vi "Drag Drop Test.vi"() -> ()   [LabVIEW 2020]
uses:
  <vilib>/picture/picture.llb/imagedata.ctl
  <vilib>/event_ctls.llb/lveventtype.ctl
panel:
  out "2D Picture 3":picture
  out "2D Picture 2":picture
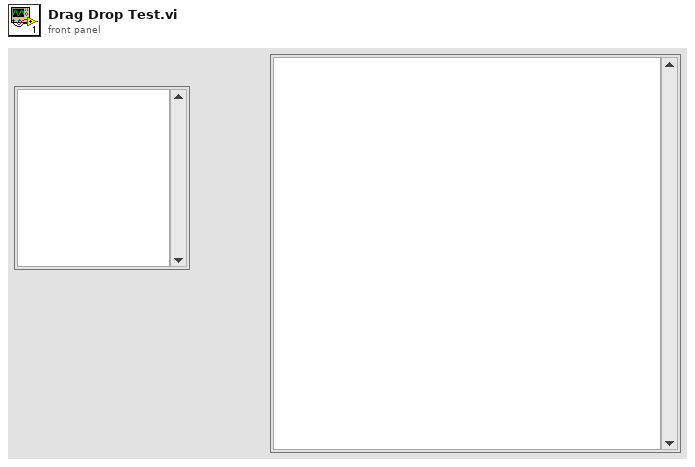
[diagram p1: front panel]
types:
  T1 = typedef "imagedata.ctl" = cluster{"image type":i32, "image depth":i32, "image":u8[], "mask":u8[], "colors":u32[], "Rectangle":cluster{"left":i16, "top":i16, "right":i16, "bottom":i16}}
  T2 = cluster{"Name":string, "CPTM.DataType":variant, "Get All Control Values Variant":cluster{"Name":string, "Variant Data":variant}[], "Color 256":T1}[]
  T3 = cluster{"left":i16, "top":i16, "right":i16, "bottom":i16}
  T4 = typedef "lveventtype.ctl" = enum32{"Null", "Timeout", "Annotation Menu Selection", "Annotation Menu Selection?", "App Instance Close", "App Instance Close?", "Autoscale Range Change", "Bookmark Info Change", "Cell Edit", "Cell Edit?", "Cursor Grab", "Cursor Grab?", "Cursor Menu Selection", "Cursor Menu Selection?", "Cursor Move", "Cursor Release", "Data Change", "Direction Change", "Display State Change", "Drag Ended", "Drag Enter", "Drag Leave", "Drag Over", "Drag Source Update", "Drag Starting", "Drag Starting?", "Drop", "Exec State Change", "Key Down", "Key Down?", "Key Repeat", "Key Repeat?", "Key Up", "Listbox Double Click", "Menu Activation?", "Menu Selection (App)", "Menu Selection? (App)", "Menu Selection (User)", "Mouse Down", "Mouse Down?", "Mouse Enter", "Mouse Leave", "Mouse Move", "Mouse Up", "Mouse Wheel", "NI Security User Change (App)", "Pane Size", "Panel Close", "Panel Close?", "Panel Resize", "Plot Attribute Change", "Scale Range Change", "Shortcut Menu Activation?", "Shortcut Menu Selection (App)", "Shortcut Menu Selection? (App)", "Shortcut Menu Selection (User)", "Tree Double Click", "Tree Drag", "Tree Drag?", "Tree Drop", "Tree Drop?", "Tree Item Close", "Tree Item Close?", "Tree Item Open", "Tree Item Open?", "User Event", "Value Change"}
  T5 = typedef "LVPoint32TypeDef.ctl" = cluster{"Horizontal":i32, "Vertical":i32}
  T6 = typedef "LVPointTypeDef.ctl" = cluster{"Horizontal":i16, "Vertical":i16}
  T7 = typedef "LVPositionTypeDef.ctl" = cluster{"Left":i32, "Top":i32}
  T8 = cluster{"Name":string, "CPTM.DataType":variant, "Get All Control Values Variant":cluster{"Name":string, "Variant Data":variant}[], "Color 256":T1}
  T9 = cluster{string, cluster{"Name":string, "Color 256":T1}}
  T10 = cluster{string, cluster{"Name":string, "Color 256":T1}}[]
  T11 = cluster{"Left":i32, "Top":i32, "Left":i32, "Top":i32}
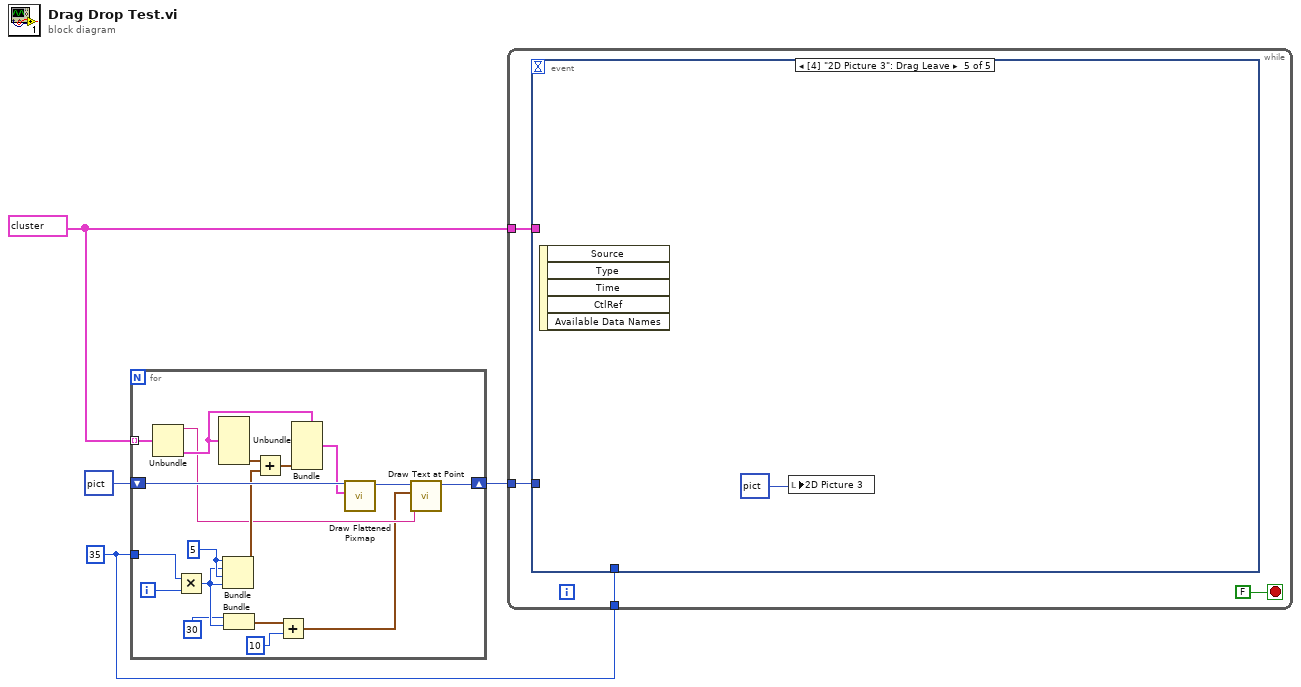
[diagram p0: block diagram]
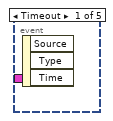
[diagram p2: hidden frame]
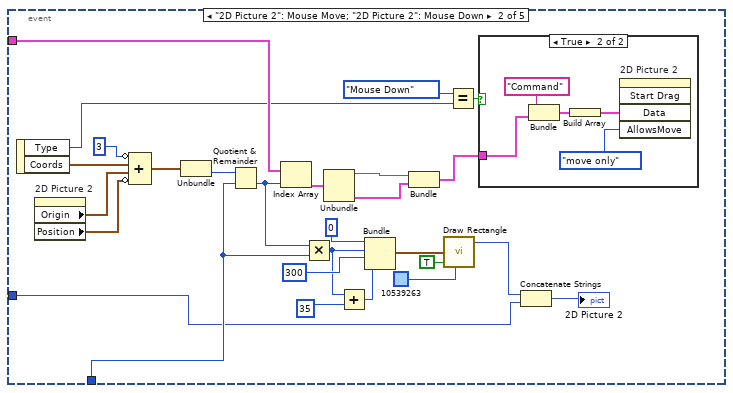
[diagram p3: hidden frame]
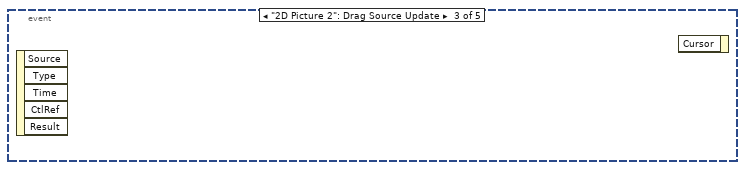
[diagram p5: hidden frame]
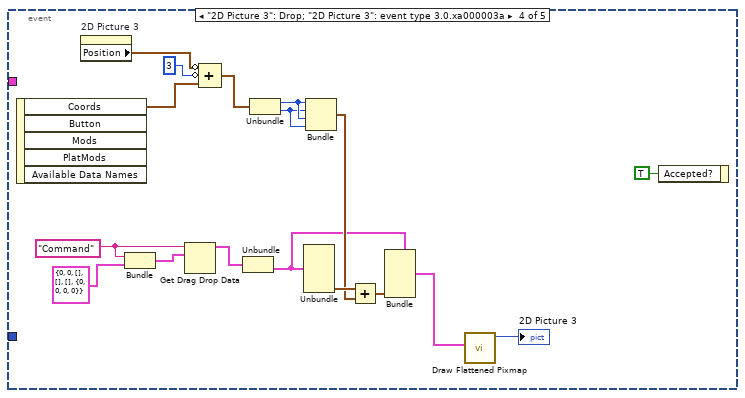
[diagram p6: hidden frame]
diagram:
  w2 = 35
  w1 = T2 data[51771B] ("Array")
  n1 = for {
    tunnel: w1 -> [w21] mode=indexing
    shift-right: [w12] -> w3
    shift-left: picture data[5B] ("2D Picture") -> [w22]
    tunnel: w2 -> [w5]
    i -> [w17]
    w16 = 5
    n2 = Unbundle(w21) -> ("Name"=w9:string, "Color 256"=w20:T1)  [unwired: 2 out]
    n3 = Multiply(x=w5, y=w17) -> (x*y=w11:i32)
    n4 = Unbundle(w20) -> ("Rectangle"=w18:T3)  [unwired: 5 out]
    n5 = Bundle(w16, w11, w16, w11) -> (w15:cluster{i32, i32, i32, i32})  [unwired: 1 in]
    n6 = Bundle(30, w11) -> (w8:cluster{i32, i32})  [unwired: 1 in]
    n7 = Add(x=w18, y=w15) -> (x+y=w14:cluster{i32, i32, i32, i32})
    n8 = Add(x=w8, y=10) -> (x+y=w7:cluster{i32, i32})
    n9 = Bundle(cluster=w20, "Rectangle"=w14) -> (w19:T1)  [unwired: 5 in]
    n10 = call <vilib>:"Draw Flattened Pixmap.vi"("image data"=w19, "picture"=w22) -> ("new picture"=w13:picture)  [unwired: 7 in]
    n11 = call <vilib>:"Draw Text at Point.vi"("text"=w9, "origin"=w7, "picture"=w13) -> ("new picture"=w12:picture)  [unwired: 7 in, 1 out]
  }
  n12 = while {
    tunnel: w3 -> [w25]
    tunnel: w2 -> [w24]
    tunnel: w1 -> [w23]
    stop <- FALSE stop-if-true
    n13 = event shown="[4] \"2D Picture 3\": Drag Leave" {
      selector: _ -> [_ _ _ _ _]
      dyn-events: _ -> [_ _ _ _ _]
      timeout: _ -> [_ _ _ _ _]
      tunnel: w25 -> [_ w36 _ _ _]
      tunnel: w24 -> [_ w45 _ _ _]
      tunnel: w23 -> [_ w47 _ _ _]
      event Timeout {
        n14 = event-data() -> ()  [unwired: 1 in, 3 out]
      }
      event "2D Picture 2": Mouse Move; "2D Picture 2": Mouse Down {
        n15 = event-data() -> ("Type"=w31:T4, "Coords"=w53:T5)  [unwired: 1 in]
        n16 = property on="2D Picture 2" class="Pict"() -> ("Origin"=w52:T6, "Position"=w51:T7)  [unwired: 2 in, 2 out]
        n17 = Compound Arithmetic op=ADD(invert 3, w53, w52, invert w51) -> (w49:T5)
        n18 = Unbundle(w49) -> ("Vertical"=w48:i32)  [unwired: 1 out]
        n19 = Quotient & Remainder(x=w48, y=w45) -> (floor(x/y)=w44:i32)  [unwired: 1 out]
        n20 = Index Array(array=w47, index=w44) -> (element=w46:T8)
        n21 = Multiply(x=w44, y=w45) -> (x*y=w41:i32)
        n22 = Unbundle(w46) -> ("Name"=w29:string, "Color 256"=w28:T1)  [unwired: 2 out]
        n23 = Add(x=w41, y=35) -> (x+y=w39:i32)
        n24 = Bundle(0, w41, 300, w39) -> (w38:cluster{i32, i32, i32, i32})  [unwired: 1 in]
        n25 = Bundle("Name"=w29, "Color 256"=w28) -> (w27:cluster{"Name":string, "Color 256":T1})  [unwired: 1 in]
        n26 = call <vilib>:"Draw Rectangle.vi"("rect"=w38, "fill?(F)"=TRUE, "color(black)"=u32 10539263) -> ("new picture"=w35:picture)  [unwired: 6 in]
        n27 = Equal?(x=lveventtype."Mouse Down" ("Type"), y=w31) -> (x = y?=w30:bool)
        n28 = case shown="True" w30 {
          tunnel: w27 -> [_ w55]
          frame False {
          }
          frame True {
            n29 = Bundle("Command", w55) -> (w56:T9)  [unwired: 1 in]
            n30 = Build Array(w56) -> (w57:T10)
            n31 = invoke on="2D Picture 2" class="Pict" method="Start Drag"("Data"=w57, "AllowsMove"=enum32{"copy or move", "copy only", "move only"}."move only" ("Drag Mode")) -> ()  [unwired: 3 in, 5 out]
          }
        }
        n32 = Concatenate Strings(w35, w36) -> (→"2D Picture 2":picture)
      }
      event "2D Picture 2": Drag Source Update {
        n33 = event-data() -> ()  [unwired: 1 in, 5 out]
        n34 = event-data() -> ()  [unwired: 2 in, 1 out]
      }
      event "2D Picture 3": Drop; "2D Picture 3": event type 3.0.xa000003a {
        w74 = "Command"
        n35 = event-data() -> ("Coords"=w62:T5)  [unwired: 1 in, 4 out]
        n36 = property on="2D Picture 3" class="Pict"() -> ("Position"=w60:T7)  [unwired: 2 in, 2 out]
        n37 = Bundle(w74, "output cluster"=T1 {"image type"=0, "image depth"=0, "image"=[], "mask"=[], "colors"=[], "Rectangle"={"left"=0, "top"=0, "right"=0, "bottom"=0}}) -> (w73:cluster{string, "output cluster":T1})  [unwired: 1 in]
        n38 = Get Drag Drop Data(8:w73, 9:w74) -> (3:w72:cluster{string, "output cluster":T1})  [unwired: 1 in, 1 out]
        n39 = Compound Arithmetic op=ADD(invert w60, invert 3, w62) -> (w61:T7)
        n40 = Unbundle(w72) -> ("output cluster"=w65:T1)  [unwired: 1 out]
        n41 = Unbundle(w61) -> ("Left"=w68:i32, "Top"=w67:i32)
        n42 = Unbundle(w65) -> ("Rectangle"=w69:T3)  [unwired: 5 out]
        n43 = Bundle("Left"=w68, "Top"=w67, "Left"=w68, "Top"=w67) -> (w66:T11)  [unwired: 1 in]
        n44 = Add(x=w69, y=w66) -> (x+y=w70:cluster{i32, i32, i32, i32})
        n45 = Bundle(cluster=w65, "Rectangle"=w70) -> (w64:T1)  [unwired: 5 in]
        n46 = call <vilib>:"Draw Flattened Pixmap.vi"("image data"=w64) -> ("new picture"=→"2D Picture 3":picture)  [unwired: 8 in]
        n47 = event-data("Accepted?"=TRUE) -> ()  [unwired: 1 in, 1 out]
      }
      event "2D Picture 3": event #0x3d {
        n48 = event-data() -> ()  [unwired: 1 in, 5 out]
        n49 = local write "2D Picture 3"(picture data[5B] ("2D Picture")) -> ()
      }
    }
  }
